vi "VoltageInputGetSensorUnit.vi"(0 "error in (no error)":errorcluster, 3 "Device In":u64) -> (7 "error out":errorcluster, 8 "Name":string, 9 "Symbol":string, 10 "Device Out":u64)   [LabVIEW 2012, in "Phidget Voltage Input.lvlib"]
doc: "${SensorUnit:Header}"
uses:
  <instrlib>/Phidgets/Phidget Voltage Input/Phidget Voltage Input.lvlib
  <vilib>/Utility/importsl/GetValueByPointer/datatype.ctl
  <vilib>/Utility/importsl/GetValueByPointer/GetValueByPointer.xnode
  <instrlib>/Phidgets/Phidget Common/Phidget Common.lvlib
  phidget22.dll
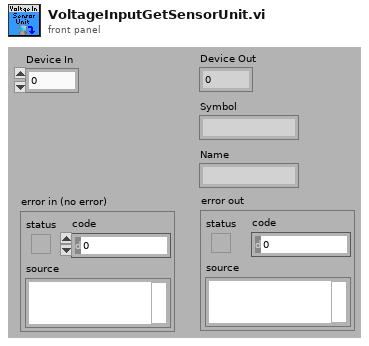
[diagram p1: front panel]
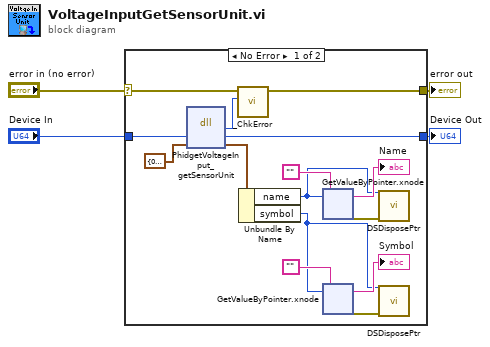
[diagram p0: block diagram]
diagram:
  n1 = case shown="No Error" "error in (no error)" {
    selector: "error in (no error)" -> [w16 w45]
    tunnel: [w15 w45] -> w3
    tunnel: "Device In" -> [w19 w44]
    tunnel: [w18 w44] -> w1
    frame No Error {
      n2 = dll-call lib="phidget22.*" fn="PhidgetVoltageInput_getSensorUnit"("phid"=w19, "unitInfo"=cluster{"unit":u32, "name":u32, "symbol":u32} {"unit"=0, "name"=0, "symbol"=0} ("sensorUnit")) -> ("return type"=w17:i32, "phid"=w18:u64, "unitInfo"=w5:cluster{"unit":u32, "name":u32, "symbol":u32})  [unwired: 3 in, 2 out]
      n3 = call <instrlib>:"_ChkError.vi"("Return Code"=w17, "error in (no error)"=w16) -> ("error out"=w15:errorcluster)  [unwired: 9 in]
      n4 = Unbundle By Name(w5) -> ("name"=w7:u32, "symbol"=w11:u32)
      n5 = xnode "GetValueByPointer.xnode"("Pointer"=w7, "InputType"="") -> ("Output"=→"Name":string, "ErrorOut"=w6:errorcluster)  [unwired: 2 in]
      n6 = xnode "GetValueByPointer.xnode"("Pointer"=w11, "InputType"="") -> ("Output"=→"Symbol":string, "ErrorOut"=w10:errorcluster)  [unwired: 2 in]
      n7 = call <vilib>:"DSDisposePtr.vi"("error in (no error)"=w6, "Pointer"=w7) -> ()  [unwired: 9 in, 1 out]
      n8 = call <vilib>:"DSDisposePtr.vi"("error in (no error)"=w10, "Pointer"=w11) -> ()  [unwired: 9 in, 1 out]
    }
    frame Error {
    }
  }
  "error out" <- w3
  "Device Out" <- w1
